vi "SpanCalibrateChannels.vi"(8 "error in":errorcluster, 11 "nScale":i32) -> (0 "error out":errorcluster, 3 "Return Code":i32)   [LabVIEW 2015]
doc: "MEScope_SpanCalChans\nDescription: \nThis function will read the ADC offset for channels 1 and 2, after first setting the hardware for the appropriate scale. The values are stored in the Local EEPROM structure.\nDetail: \nint MEScope_SpanCalChans (\nint nScale \n);\n\nParameters:\nint nScale - which scale to use (CHANNEL_SCALE_1V to CHANNEL_SCALE_400V)\n\nReturn Values:\nThis function returns a 0 if the function completed successfully. A non-zero return code will indicate error.\nRemarks:\nScale definitions:\n#define CHANNEL_SCALE_1V 0\n#define CHANNEL_SCALE_2V 1\n#define CHANNEL_SCALE_5V 2\n#define CHANNEL_SCALE_10V 3\n#define CHANNEL_SCALE_20V 4\n#define CHANNEL_SCALE_50V 5\n#define CHANNEL_SCALE_100V 6\n#define CHANNEL_SCALE_200V 7\n#define CHANNEL_SCALE_400V 8\nSerial Command packet: \nn/a"
uses:
  ScannerDiagDLL.dll
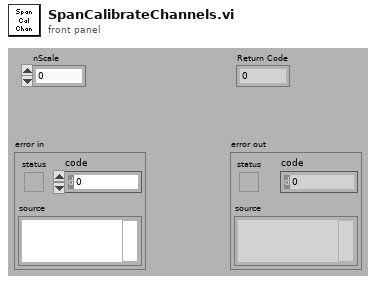
[diagram p1: front panel]
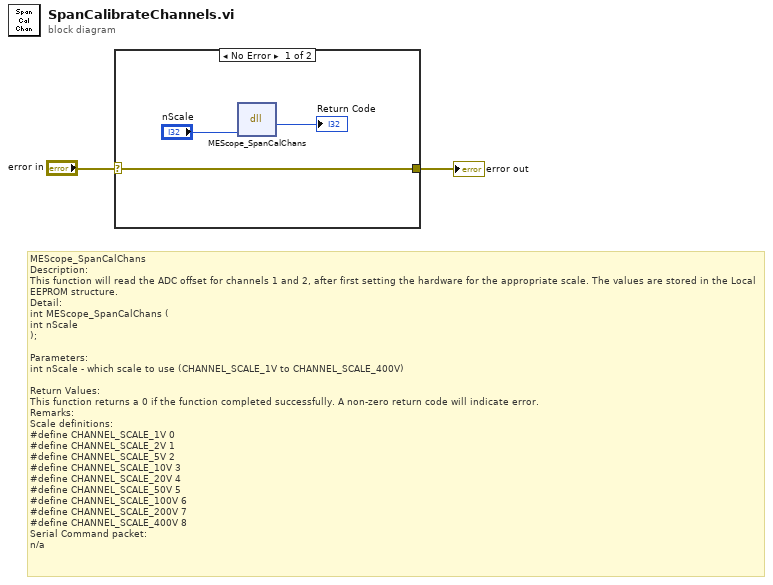
[diagram p0: block diagram]
diagram:
  # "MEScope_SpanCalChans\nDescription: \nThis function will read the ADC offset for channels 1 and 2, after first setting the hardware for the appropriate scale. The values are stored in the Local EEPROM structure.\nDetail: \nint MEScope_SpanCalChans (\nint nScale \n);\n\nParameters:\nint nScale - which scale to use (CHANNEL_SCALE_1V to CHANNEL_SCALE_400V)\n\nReturn Values:\nThis function returns a 0 if the function completed successfully. A non-zero return code will indicate error.\nRemarks:\nScale definitions:\n#define CHANNEL_SCALE_1V\t0\n#define CHANNEL_SCALE_2V\t1\n#define CHANNEL_SCALE_5V\t2\n#define CHANNEL_SCALE_10V\t3\n#define CHANNEL_SCALE_20V\t4\n#define CHANNEL_SCALE_50V\t5\n#define CHANNEL_SCALE_100V\t6\n#define CHANNEL_SCALE_200V\t7\n#define CHANNEL_SCALE_400V\t8\nSerial Command packet: \nn/a"
  n1 = case shown="No Error" "error in" {
    selector: "error in" -> [w4 w6]
    tunnel: [w4 w6] -> w1
    frame No Error {
      n2 = dll-call lib="C:/SNAPON/ModisEdge/TabletScope/Test Sequence/Code Modules/DLL/ScannerDiagDLL.dll" fn="MEScope_SpanCalChans" ("TripoliDLL.dll:Test_WirelessLANPort")("nScale"="nScale") -> ("return type"=→"Return Code":i32)  [unwired: 4 in, 2 out]
    }
    frame Error {
    }
  }
  "error out" <- w1
